vi "Destroy Broadcast Events.vi"(8 "error in":errorcluster) -> (0 "error out":errorcluster)   [LabVIEW 2024, in "Sing.lvlib"]
doc: "Destroy the broadcast events, even if there is an incoming error.\n\n<b>NOTE</b>: The contents of this VI are automatically generated and modified by the <b>Tools > DQMH Consortium > DQMH</b> utilities. Consider using those utilities instead of making your own modifications to this VI.\n_____\nBased on DQMH Dev Tools: Project Template 7.1.0.1503."
uses:
  Sing.lvlib
panel:
  # "NOTE: The contents of this VI are automatically generated and modified by the Tools > DQMH Consortium > DQMH utilities. Consider using those utilities instead of making your own modifications to this VI."
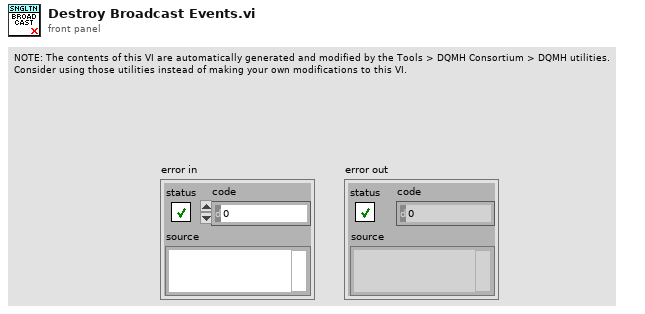
[diagram p1: front panel]
types:
  T1 = typedef "Sing.lvlib/Broadcast Events--cluster.ctl" = cluster{"Module Did Init":refnum<user-event>, "Status Updated":refnum<user-event>, "Error Reported":refnum<user-event>, "Did Something":refnum<user-event>, "Module Did Stop":refnum<user-event>, "Update Module Execution Status":refnum<user-event>}
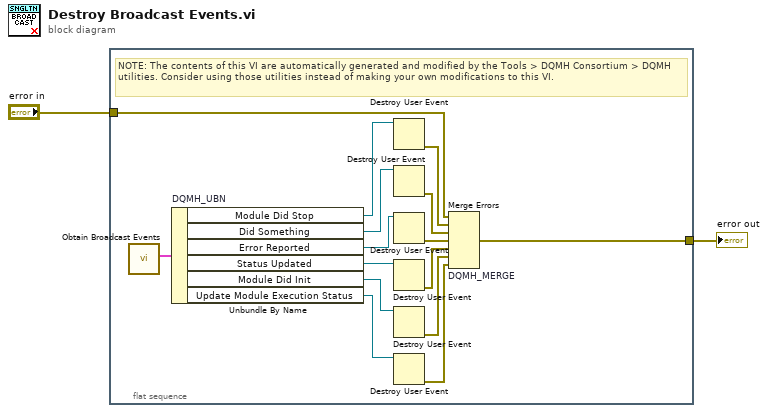
[diagram p0: block diagram]
diagram:
  n1 = flat-sequence {
    tunnel: [w16] -> w2
    tunnel: "error in" -> [w5]
    frame #0 {
      # "NOTE: The contents of this VI are automatically generated and modified by the Tools > DQMH Consortium > DQMH utilities. Consider using those utilities instead of making your own modifications to this VI."
      n2 = call "Obtain Broadcast Events.vi"() -> ("Sing Broadcast Events"=w15:T1)  [unwired: 10 in, 1 out]
      n3 = Unbundle By Name "DQMH_UBN"(w15) -> ("Module Did Stop"=w6:refnum<user-event>, "Did Something"=w9:refnum<user-event>, "Error Reported"=w10:refnum<user-event>, "Status Updated"=w13:refnum<user-event>, "Module Did Init"=w14:refnum<user-event>, "Update Module Execution Status"=w3:refnum<user-event>)
      n4 = Destroy User Event(user event=w6) -> (error out=w7:errorcluster)  [unwired: 1 in]
      n5 = Destroy User Event(user event=w9) -> (error out=w8:errorcluster)  [unwired: 1 in]
      n6 = Destroy User Event(user event=w10) -> (error out=w11:errorcluster)  [unwired: 1 in]
      n7 = Destroy User Event(user event=w13) -> (error out=w12:errorcluster)  [unwired: 1 in]
      n8 = Destroy User Event(user event=w14) -> (error out=w17:errorcluster)  [unwired: 1 in]
      n9 = Destroy User Event(user event=w3) -> (error out=w4:errorcluster)  [unwired: 1 in]
      n10 = Merge Errors "DQMH_MERGE"(w5, w7, w8, w11, w12, w17, w4) -> (w16:errorcluster)
    }
  }
  "error out" <- w2
